vi "pulse_generator_data_v2.vi"(3 "PG Data":refnum<vi>, 4 "Record dP Data":refnum<vi>, 5 "queue in":refnum<queue>, 6 "Stop! Refnum":refnum<vi>, 7 "Recording Progressbar":refnum<vi>, 8 "Seesion Start Time":timestamp, 9 "Pulse Generator Chart Refnums":T3, 10 "Pulse Generator Offsets and Data Saving Controls Refnums":T2, 11 "Pulse Generator Measurement Refnums":T1) -> ()   [LabVIEW 2017]
uses:
  pulse_generator_data_charts_refnums.ctl
  pulse_generator_data_controls_refnums.ctl
  pulse_generator_data_refnums.ctl
  <vilib>/Waveform/WDTOps.llb/WDT Get Waveform Time Array DBL.vi
panel:
  out "size(s)":i32[](graph)
  out "Sampling Rate":refnum<vi>
  out "Recording Duration":refnum<vi>
  out "Camera Voltage Chart":refnum<vi>
  out "Abs Tank Pressure Chart":refnum<vi>
  out "Pitot dP Chart":refnum<vi>
  out "Pulse Generator to Test Section dP Chart":refnum<vi>
  out "W1-7 dP":refnum<vi>
  out "W1-4 dP":refnum<vi>
  out "Mass Flow Rate":refnum<vi>
  out "Liquid Sat Pressure":refnum<vi>
  out "Liquid Temperature":refnum<vi>
  out "Vapor Sat Pressure":refnum<vi>
  out "Vapor Temperature":refnum<vi>
  out "Pitot dP":refnum<vi>
  out "PG to TS dP":refnum<vi>
  out "Pitot Current":refnum<vi>
  out "PG Abs Pressure":refnum<vi>
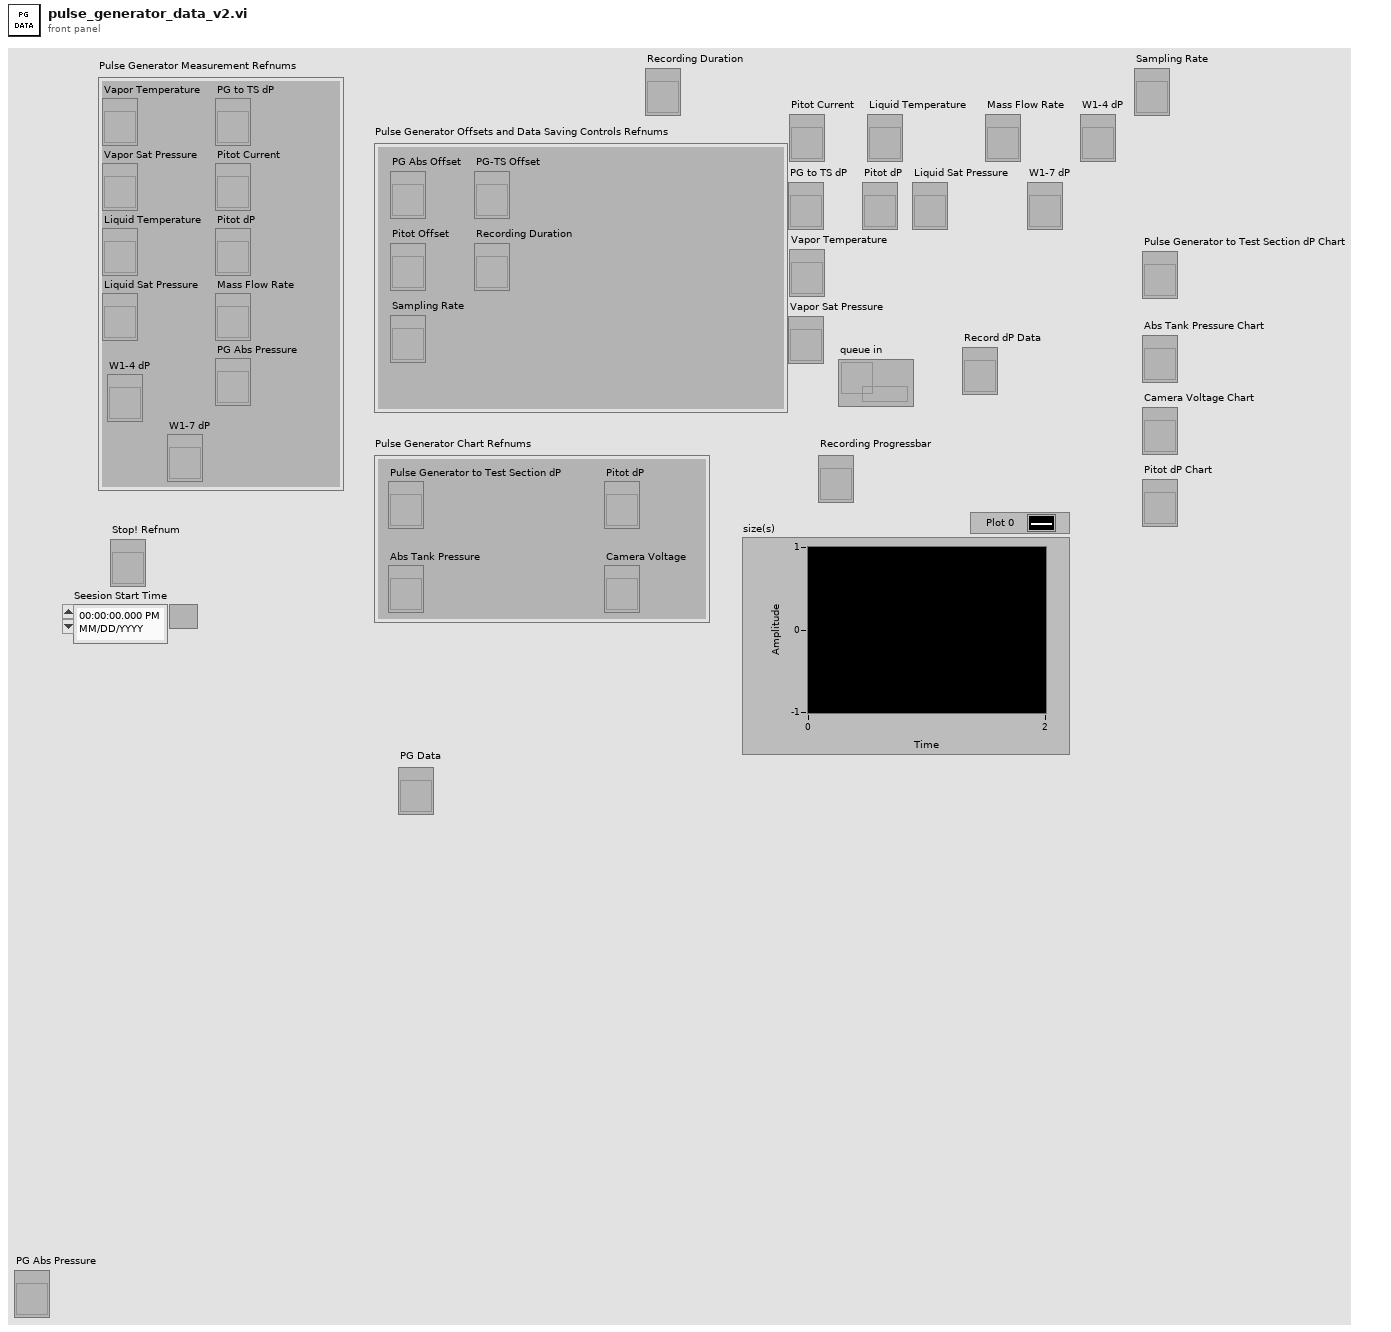
[diagram p1: front panel]
types:
  T1 = typedef "pulse_generator_data_refnums.ctl" = cluster{"Vapor Temperature":refnum<vi>, "Vapor Sat Pressure":refnum<vi>, "Liquid Temperature":refnum<vi>, "Liquid Sat Pressure":refnum<vi>, "PG to TS dP":refnum<vi>, "Pitot Current":refnum<vi>, "Pitot dP":refnum<vi>, "Mass Flow Rate":refnum<vi>, "PG Abs Pressure":refnum<vi>, "W1-4 dP":refnum<vi>, "W1-7 dP":refnum<vi>}
  T2 = typedef "pulse_generator_data_controls_refnums.ctl" = cluster{"PG Abs Offset":refnum<vi>, "Pitot Offset":refnum<vi>, "PG-TS Offset":refnum<vi>, "Recording Duration":refnum<vi>, "Sampling Rate":refnum<vi>}
  T3 = typedef "pulse_generator_data_charts_refnums.ctl" = cluster{"Pulse Generator to Test Section dP":refnum<vi>, "Pitot dP":refnum<vi>, "Abs Tank Pressure":refnum<vi>, "Camera Voltage":refnum<vi>}
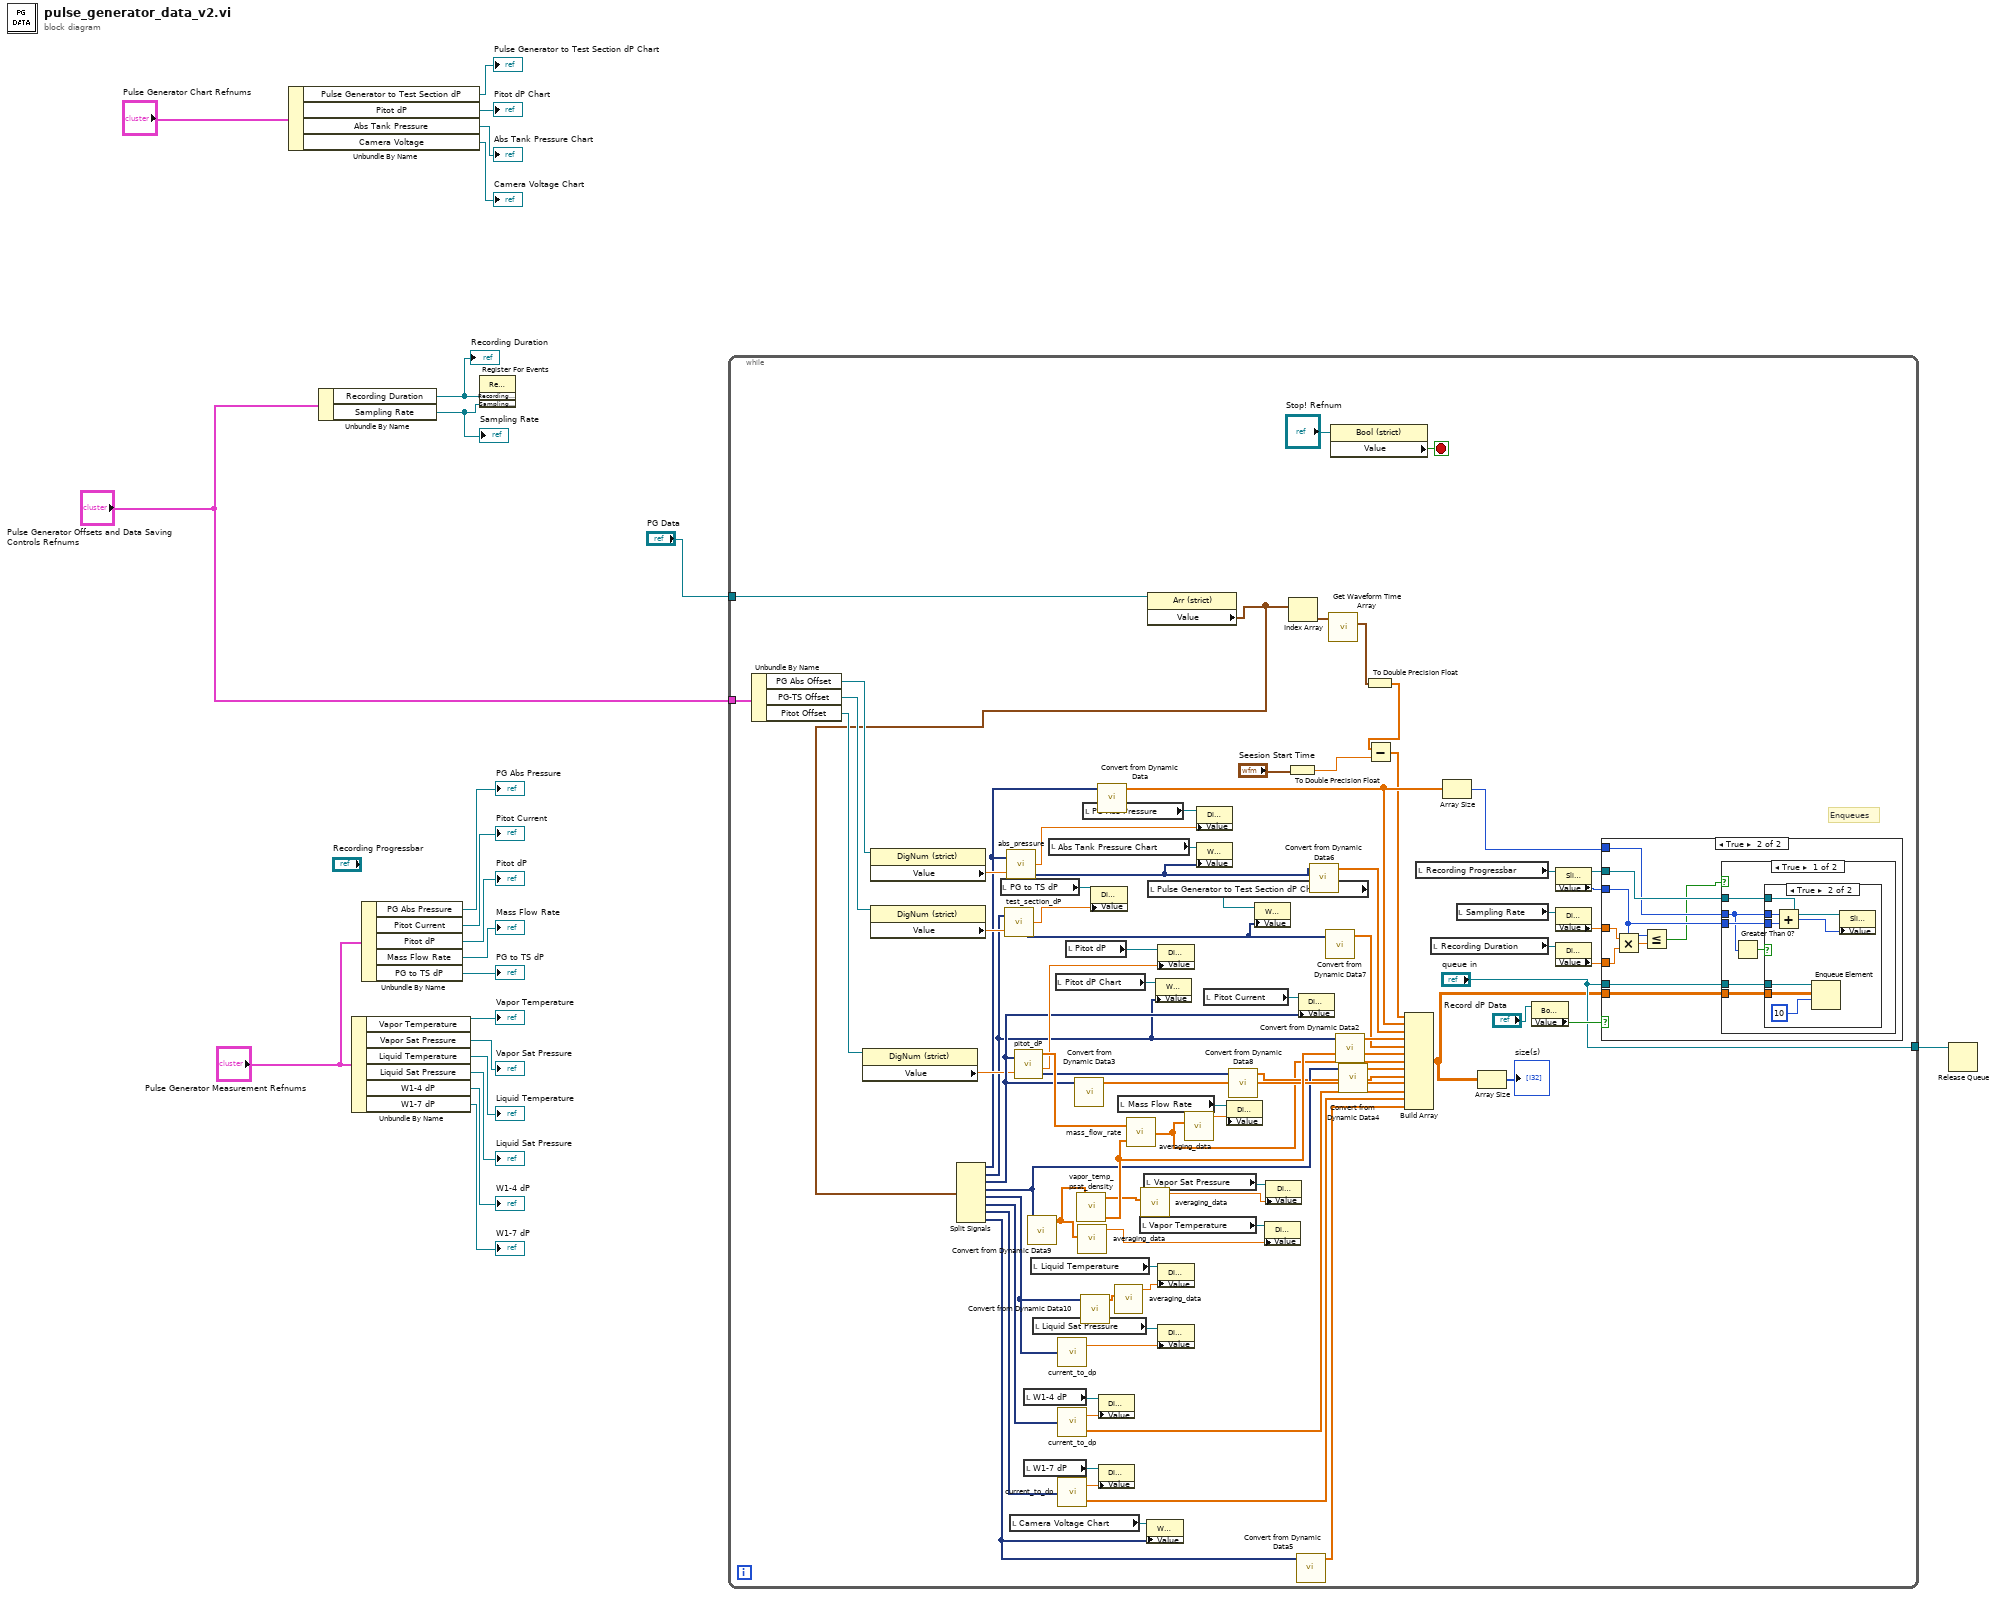
[diagram p0: block diagram]
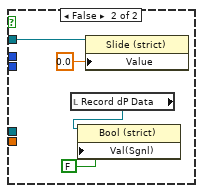
[diagram p4: hidden frame]
diagram:
  n1 = Unbundle By Name("Pulse Generator Chart Refnums") -> ("Pulse Generator to Test Section dP"=→"Pulse Generator to Test Section dP Chart":refnum<vi>, "Pitot dP"=→"Pitot dP Chart":refnum<vi>, "Abs Tank Pressure"=→"Abs Tank Pressure Chart":refnum<vi>, "Camera Voltage"=→"Camera Voltage Chart":refnum<vi>)
  n2 = Unbundle By Name("Pulse Generator Offsets and Data Saving Controls Refnums") -> ("Recording Duration"=w4:refnum<vi>, "Sampling Rate"=w3:refnum<vi>)
  "Recording Duration" <- w4
  "Sampling Rate" <- w3
  n3 = Unbundle By Name("Pulse Generator Measurement Refnums") -> ("Vapor Temperature"=→"Vapor Temperature":refnum<vi>, "Vapor Sat Pressure"=→"Vapor Sat Pressure":refnum<vi>, "Liquid Temperature"=→"Liquid Temperature":refnum<vi>, "Liquid Sat Pressure"=→"Liquid Sat Pressure":refnum<vi>, "W1-4 dP"=→"W1-4 dP":refnum<vi>, "W1-7 dP"=→"W1-7 dP":refnum<vi>)
  n4 = Unbundle By Name("Pulse Generator Measurement Refnums") -> ("PG Abs Pressure"=→"PG Abs Pressure":refnum<vi>, "Pitot Current"=→"Pitot Current":refnum<vi>, "Pitot dP"=→"Pitot dP":refnum<vi>, "Mass Flow Rate"=→"Mass Flow Rate":refnum<vi>, "PG to TS dP"=→"PG to TS dP":refnum<vi>)
  n5 = register-events(w4, w3) -> ()  [unwired: 2 in, 2 out]
  n6 = while {
    tunnel: "Pulse Generator Offsets and Data Saving Controls Refnums" -> [w102]
    tunnel: ["queue in"] -> w6
    tunnel: "PG Data" -> [w33]
    stop <- w103 stop-if-true
    # "Enqueues"
    n7 = Unbundle By Name(w102) -> ("PG Abs Offset"=w101:refnum<vi>, "PG-TS Offset"=w100:refnum<vi>, "Pitot Offset"=w99:refnum<vi>)
    n8 = property class="DigNum (strict)"(reference=w99) -> ("Value"=w51:dbl)  [unwired: 1 in, 2 out]
    n9 = property class="DigNum (strict)"(reference=w101) -> ("Value"=w98:dbl)  [unwired: 1 in, 2 out]
    n10 = property class="DigNum (strict)"(reference=w100) -> ("Value"=w55:dbl)  [unwired: 1 in, 2 out]
    n11 = local read "PG to TS dP"() -> (w97:refnum<vi>)
    n12 = local read "Camera Voltage Chart"() -> (w77:refnum<vi>)
    n13 = local read "W1-4 dP"() -> (w87:refnum<vi>)
    n14 = local read "W1-7 dP"() -> (w84:refnum<vi>)
    n15 = local read "Liquid Temperature"() -> (w90:refnum<vi>)
    n16 = local read "Liquid Sat Pressure"() -> (w92:refnum<vi>)
    n17 = local read "Abs Tank Pressure Chart"() -> (w80:refnum<vi>)
    n18 = local read "Pitot dP Chart"() -> (w79:refnum<vi>)
    n19 = local read "Pitot dP"() -> (w95:refnum<vi>)
    n20 = local read "PG Abs Pressure"() -> (w53:refnum<vi>)
    n21 = local read "Mass Flow Rate"() -> (w93:refnum<vi>)
    n22 = local read "Vapor Temperature"() -> (w89:refnum<vi>)
    n23 = local read "Vapor Sat Pressure"() -> (w82:refnum<vi>)
    n24 = property class="Arr (strict)"(reference=w33) -> ("Value"=w32:waveform(dbl)[])  [unwired: 1 in, 2 out]
    n25 = Split Signals(w32) -> (w40:dynamicdata, w49:dynamicdata, w58:dynamicdata, w56:dynamicdata, w27:dynamicdata, w86:dynamicdata, w85:dynamicdata, w67:dynamicdata)  [unwired: 8 in]
    n26 = call "test_section_dP.vi"("dP Voltage"=w49, "Offset[Pa]"=w55) -> ("Adj dP"=w75:dbl, "Adj dP Array"=w43:dynamicdata)  [unwired: 1 out]
    n27 = call "abs_pressure.vi"("Input Voltage"=w40, "Offset[Pa]"=w98) -> ("Adj Absolute Pressure"=w76:dbl, "Adj Absolute Pressure Array"=w45:dynamicdata)  [unwired: 1 out]
    n28 = call "pitot_dP.vi"("Pitot Current"=w58, "Pitot Offset [Pa]"=w51) -> ("dP H2O"=w94:dbl[], "Adj dP [Pa]"=w78:dbl, "Adj dP [Pa] Array"=w41:dynamicdata)  [unwired: 1 out]
    n29 = call "Convert from Dynamic Data9"("Dynamic Data Type"=w56) -> ("Array"=w31:dbl[])  [unwired: 3 in]
    n30 = call "current_to_dp.vi"("Current [A]"=w27) -> ("dP [Pa]"=w91:dbl)  [unwired: 1 out]
    n31 = call "current_to_dp.vi"("Current [A]"=w86) -> ("dP [Pa]"=w88:dbl, "dP Array [Pa]"=w73:dbl[])
    n32 = call "current_to_dp.vi"("Current [A]"=w85) -> ("dP [Pa]"=w83:dbl, "dP Array [Pa]"=w57:dbl[])
    n33 = call "Convert from Dynamic Data3"("Dynamic Data Type"=w58) -> ("Array"=w70:dbl[])  [unwired: 3 in]
    n34 = call "vapor_temp_psat_density.vi"("Vapor Temp [C]"=w31) -> ("Psat Vapor"=w29:dbl[], "Vapor Density"=w74:dbl[])  [unwired: 1 in]
    n35 = call "averaging_data.vi"("Input"=w31) -> ("Average"=w30:dbl)  [unwired: 5 in, 2 out]
    n36 = call "Convert from Dynamic Data10"("Dynamic Data Type"=w27) -> ("Array"=w26:dbl[])  [unwired: 3 in]
    n37 = property class="DigNum (strict)"(reference=w97, "Value"=w75) -> ()  [unwired: 1 in, 2 out]
    n38 = call "Convert from Dynamic Data"("Dynamic Data Type"=w40) -> ("Array"=w66:dbl[])  [unwired: 3 in]
    n39 = property class="DigNum (strict)"(reference=w87, "Value"=w88) -> ()  [unwired: 1 in, 2 out]
    n40 = property class="DigNum (strict)"(reference=w84, "Value"=w83) -> ()  [unwired: 1 in, 2 out]
    n41 = call "averaging_data.vi"("Input"=w26) -> ("Average"=w25:dbl)  [unwired: 5 in, 2 out]
    n42 = call "mass_flow_rate.vi"("Density"=w74, "dP H2O"=w94) -> ("Mass Flow Rate [g/s] Array"=w24:dbl[])
    n43 = call "averaging_data.vi"("Input"=w29) -> ("Average"=w28:dbl)  [unwired: 5 in, 2 out]
    n44 = property class="WFChart (strict)"(reference=w77, "Value"=w67) -> ()  [unwired: 1 in, 2 out]
    n45 = local read "Pulse Generator to Test Section dP Chart"() -> (w81:refnum<vi>)
    n46 = property class="WFChart (strict)"(reference=w79, "Value"=w49) -> ()  [unwired: 1 in, 2 out]
    n47 = property class="DigNum (strict)"(reference=w95, "Value"=w78) -> ()  [unwired: 1 in, 2 out]
    n48 = property class="DigNum (strict)"(reference=w90, "Value"=w25) -> ()  [unwired: 1 in, 2 out]
    n49 = property class="DigNum (strict)"(reference=w92, "Value"=w91) -> ()  [unwired: 1 in, 2 out]
    n50 = call "averaging_data.vi"("Input"=w24) -> ("Average"=w23:dbl)  [unwired: 5 in, 2 out]
    n51 = property class="DigNum (strict)"(reference=w53, "Value"=w76) -> ()  [unwired: 1 in, 2 out]
    n52 = property class="WFChart (strict)"(reference=w80, "Value"=w45) -> ()  [unwired: 1 in, 2 out]
    n53 = local read "Pitot Current"() -> (w96:refnum<vi>)
    n54 = property class="DigNum (strict)"(reference=w93, "Value"=w23) -> ()  [unwired: 1 in, 2 out]
    n55 = call "Convert from Dynamic Data8"("Dynamic Data Type"=w41) -> ("Array"=w42:dbl[])  [unwired: 3 in]
    n56 = property class="WFChart (strict)"(reference=w81, "Value"=w43) -> ()  [unwired: 1 in, 2 out]
    n57 = property class="DigNum (strict)"(reference=w89, "Value"=w30) -> ()  [unwired: 1 in, 2 out]
    n58 = property class="DigNum (strict)"(reference=w82, "Value"=w28) -> ()  [unwired: 1 in, 2 out]
    n59 = To Double Precision Float(number="Seesion Start Time") -> (double precision float=w35:dbl)
    n60 = Index Array(array=w32) -> (element=w39:waveform(dbl))  [unwired: 1 in]
    n61 = call "Convert from Dynamic Data5"("Dynamic Data Type"=w67) -> ("Array"=w68:dbl[])  [unwired: 3 in]
    n62 = property class="DigNum (strict)"(reference=w96, "Value"=w58) -> ()  [unwired: 1 in, 2 out]
    n63 = call "Convert from Dynamic Data6"("Dynamic Data Type"=w45) -> ("Array"=w46:dbl[])  [unwired: 3 in]
    n64 = call "Convert from Dynamic Data7"("Dynamic Data Type"=w43) -> ("Array"=w44:dbl[])  [unwired: 3 in]
    n65 = call-poly <vilib>:"Get Waveform Time Array.vi"("waveform in"=w39) -> ("X array"=w38:timestamp[])  [unwired: 9 in, 1 out]
    n66 = property class="Bool (strict)"(reference="Stop! Refnum") -> ("Value"=w103:bool)  [unwired: 1 in, 2 out]
    n67 = call "Convert from Dynamic Data2"("Dynamic Data Type"=w49) -> ("Array"=w71:dbl[])  [unwired: 3 in]
    n68 = call "Convert from Dynamic Data4"("Dynamic Data Type"=w56) -> ("Array"=w69:dbl[])  [unwired: 3 in]
    n69 = To Double Precision Float(number=w38) -> (double precision float=w37:dbl[])
    n70 = Subtract(x=w37, y=w35) -> (x-y=w34:dbl[])
    n71 = Build Array(w34, w66, w46, w71, w44, w74, w24, w69, w42, w70, w73, w57, w68) -> (w48:dbl[][])
    n72 = local read "Recording Progressbar"() -> (w60:refnum<vi>)
    n73 = local read "Recording Duration"() -> (w64:refnum<vi>)
    n74 = Array Size(array=w66) -> (size(s)=w52:i32)
    n75 = local read "Sampling Rate"() -> (w65:refnum<vi>)
    n76 = Array Size(array=w48) -> (size(s)=→"size(s)":i32[])
    n77 = property class="Bool (strict)"(reference="Record dP Data") -> ("Value"=w54:bool)  [unwired: 1 in, 2 out]
    n78 = property class="Slide (strict)"(reference=w60) -> (reference out=w59:refnum<vi>, "Value"=w61:u32)  [unwired: 1 in, 1 out]
    n79 = property class="DigNum (strict)"(reference=w65) -> ("Value"=w63:dbl)  [unwired: 1 in, 2 out]
    n80 = property class="DigNum (strict)"(reference=w64) -> ("Value"=w62:dbl)  [unwired: 1 in, 2 out]
    n81 = case shown="True" w54 {
      tunnel: "queue in" -> [_ w113]
      tunnel: w52 -> [_ w106]
      tunnel: w63 -> [_ w112]
      tunnel: w62 -> [_ w111]
      tunnel: w61 -> [_ w109]
      tunnel: w59 -> [_ w108]
      tunnel: w48 -> [_ w107]
      frame False {
      }
      frame True {
        n82 = Multiply(x=w112, y=w111) -> (x*y=w110:dbl)
        n83 = Less Or Equal?(x=w109, y=w110) -> (x <= y?=w105:bool)
        n84 = case shown="True" w105 {
          tunnel: w113 -> [w119 _]
          tunnel: w108 -> [w118 w130]
          tunnel: w109 -> [w117 _]
          tunnel: w106 -> [w114 _]
          tunnel: w107 -> [w116 _]
          frame True {
            n85 = Greater Than 0?(x=w114) -> (x > 0?=w115:bool)
            n86 = case shown="True" w115 {
              tunnel: w119 -> [_ w125]
              tunnel: w118 -> [_ w124]
              tunnel: w117 -> [_ w122]
              tunnel: w114 -> [_ w121]
              tunnel: w116 -> [_ w120]
              frame False {
              }
              frame True {
                n87 = Add(x=w121, y=w122) -> (x+y=w123:u32)
                n88 = Enqueue Element(queue=w125, element=w120, timeout in ms (-1)=10) -> ()  [unwired: 1 in, 3 out]
                n89 = property class="Slide (strict)"(reference=w124, "Value"=w123) -> ()  [unwired: 1 in, 2 out]
              }
            }
          }
          frame False {
            n90 = local read "Record dP Data"() -> (w127:refnum<vi>)
            n91 = property class="Bool (strict)"(reference=w127, "Val(Sgnl)"=FALSE ("Value (Signaling)")) -> ()  [unwired: 1 in, 2 out]
            n92 = property class="Slide (strict)"(reference=w130, "Value"=0.0) -> ()  [unwired: 1 in, 2 out]
          }
        }
      }
    }
  }
  n93 = Release Queue(queue=w6) -> ()  [unwired: 2 in, 3 out]
